vi "SYST_ERR_COUN.vi"(0 "VISA IN":refnum<visa-resource-name>, 5 "error in":errorcluster) -> (14 "VISA Out":refnum<visa-resource-name>, 16 "Data":string, 19 "error out":errorcluster)   [LabVIEW 2018, in "PNA-X.lvlib"]
doc: "SYSTem:ERRor:COUNt? \n1874\n\n(Read-only) Returns the number of errors in the error queue. Use SYST:ERR? to read an error. \nExamples SYST:ERR:COUN? \nsystem:error:count? \nDefault Not Applicable"
uses:
  PNA-X.lvlib
panel:
  in  "Cmdline":string="SYSTem:ERRor:COUNt? "
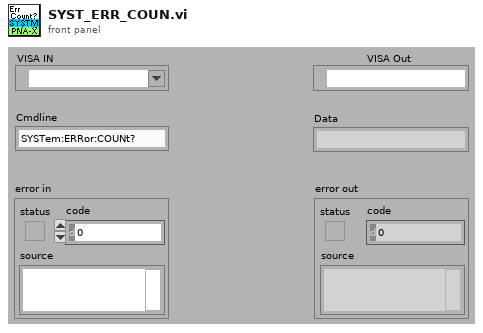
[diagram p1: front panel]
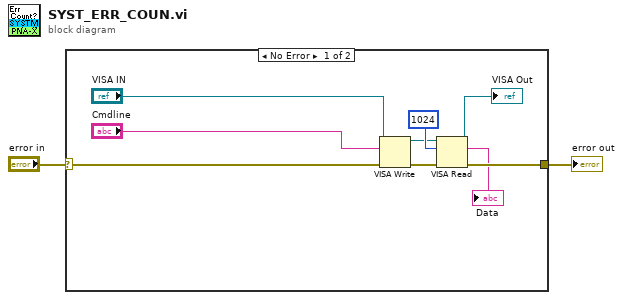
[diagram p0: block diagram]
diagram:
  n1 = case shown="No Error" "error in" {
    selector: "error in" -> [w3 w12]
    tunnel: [w7 w12] -> w1
    frame No Error {
      n2 = VISA Write(VISA resource name="VISA IN", write buffer="Cmdline", error in (no error)=w3) -> (VISA resource name out=w8:refnum<visa-resource-name>, error out=w10:errorcluster)  [unwired: 1 out]
      n3 = VISA Read(VISA resource name=w8, byte count=1024, error in (no error)=w10) -> (VISA resource name out=→"VISA Out":refnum<visa-resource-name>, read buffer=→"Data":string, error out=w7:errorcluster)  [unwired: 1 out]
    }
    frame Error {
    }
  }
  "error out" <- w1
